vi "Main Output Messages.vi"(8 "error in (no error)":errorcluster, 11 "J1939 Main Configuration":T1={"Parameters"={"J1939 XNET Settings"={"XNET Database"="", "XNET Cluster"="", "CAN Port"="", "Baud rate [Bd]"=0, "Termination"=0, "Incoming Rate"=0, "Outcoming Rate"=1, "Write Decimation"=1}, "Incoming Single Point Configuraiton"={"Incoming Single Point Frame"={"ID"=[], "Conversion"=[], "Channel Array Positions"=[], "Frame Length"=[]}, "Channel Pairs"={"Chan Refs"=[], "Previous Chan Values"=[]}, "Read FIFO"=refnum}, "Outgoing Cyclic Configuraiton"={"Outgoing Cyclic Frame"={"ID"=[], "Conversion"=[], "Channel Array Positions"=[], "Frame Length"=[], "Transmit Propreties"=[]}, "Channel Pairs"={"Block Data Refs"=[], "Previous Chan Values"=[]}, "Write FIFO"=refnum}, "J1939 Monitor Settings"={"J1939 Network Address"=0, "Name"=0}, "Simulated Addresses"=[], "Simulated Addresses LUT"=variant, "Name"=""}, "Name"="", "J1939 Cluster"={"Processed Incoming"=refnum, "Current Device Address"=0, "Processed Outgoing"=refnum, "Process Outgoing"=refnum, "Name"=0}, "References"={"BAM Buffer"=refnum, "CM Buffer"=refnum, "CM Gen"=refnum, "BAM Gen"=refnum, "Address Claims"=refnum, "RQST"=refnum}, "Frame In"="", "Frame Out"="", "Incoming Timeout"=0, "Outgoing Timeout"=0, "Listener ID"=refnum, "Process"=refnum, "Data Ref"=refnum, "Scale Ref"=refnum, "Incoming Direct Access"={"Offset"=0, "Length"=0}, "Outgoing Direct Access"={"Offset"=0, "Length"=0}, "TCP Mngr Ref"=refnum, "Name and Address"="", "Simulated Addresses"=[], "Simulated Addresses LUT"=variant} {"Simulated Addresses"."Simulated Addresses"."J1939 XNET Settings"."Name" format="%.0x"; "Simulated Addresses"."Simulated Addresses"."DM1 Data"."Data Reference" format="%.0x"; "Simulated Addresses"."Simulated Addresses"."DM1 Enable?"."Data Reference" format="%.0x"; "Simulated Addresses"."Simulated Addresses"."DM2 Data"."Data Reference" format="%.0x"; "Simulated Addresses"."Simulated Addresses"."DM2 Enable?"."Data Reference" format="%.0x"; "Parameters"."Simulated Addresses"."Simulated Addresses"."J1939 XNET Settings"."Name" format="%.0x"; "Parameters"."J1939 Monitor Settings"."Name" format="%.0x"; "Parameters"."Outgoing Cyclic Configuraiton"."Channel Pairs"."Block Data Refs"."Data Reference" format="%.0x"; "Parameters"."Outgoing Cyclic Configuraiton"."Outgoing Cyclic Frame"."Transmit Propreties"."Transmit Time" format="%#_p"; "Parameters"."J1939 XNET Settings"."Termination" items=["Off", "On"]; "Parameters"."Incoming Single Point Configuraiton"."Channel Pairs"."Chan Refs" format="%.0x"}) -> (0 "error out":errorcluster)   [LabVIEW 2015, in "J1939 Addon Engine.lvlib"]
uses:
  J1939 Addon Engine.lvlib
  Types/Configuration Cluster.ctl
  <vilib>/NI/NI VeriStand Inline Async API/_VS Inline Async API/Process/Process.lvclass
  Types/Process Parameters.ctl
  Shared/Types/XNET Settings.ctl
  Types/Incoming Single Point Configuration.ctl
  Types/Incoming Single Point Frame Pairs.ctl
  Types/Incoming Single Point Channel Pairs.ctl
  <vilib>/NI Veristand/Custom Device API/Data Reference.ctl
  Types/Outgoing Cyclic Configuration.ctl
  Types/Outgoing Cyclic Frame Pairs.ctl
  Shared/Types/XNET Frame Event Properties.ctl
  Types/Outgoing Cyclic Channel Pairs.ctl
  <vilib>/NI Veristand/Custom Device API/Block Data Reference.ctl
  Shared/Types/Monitor Settings.ctl
  Types/Simulated Settings.ctl
  Shared/Types/Compiled Simulated Settings.ctl
  Types/DTC FIFOs.ctl
  Shared/J1939 Multi Packet Frame/Types/Setup Information Cluster.ctl
  <vilib>/xnet/xnet.llb/XNET Frame CAN.ctl
  <vilib>/xnet/xnet.llb/XNET Frame Type CAN.ctl
  Shared/J1939 Utilities/Types/CAN Outgoing Message Cluster.ctl
  Shared/J1939 Multi Packet Frame/Types/TP List References.ctl
  Shared/J1939 Multi Packet Frame/Types/BAM Buffer Connections List_Ref.ctl
  Shared/J1939 Multi Packet Frame/Types/TP Buffer Connection Cluster.ctl
  Shared/J1939 Multi Packet Frame/Types/Connection Mode Generation Connection Ref.ctl
  Shared/J1939 Multi Packet Frame/Types/Connection Mode Generation Connection Cluster.ctl
  Shared/J1939 Multi Packet Frame/Types/BAM Generation Connections List_Ref.ctl
  Shared/J1939 Multi Packet Frame/Types/BAM Generation Connection Cluster.ctl
  Shared/J1939 Multi Packet Frame/Types/Address Table Reference.ctl
  Shared/J1939 Multi Packet Frame/Types/RQST Lookup Table Reference.ctl
  Types/Data Lookup Table Reference.ctl
  Types/Datatable Lookup DVR.ctl
  Types/Conversion Lookup Table Reference.ctl
  Shared/J1939 Multi Packet Frame/Types/RQST Comm Lookup Table_Ref.ctl
  Shared/STM/Connection Manager/stm_ManagerStateVariables.ctl
  Shared/STM/TCP/stm_TCP Connection Info.ctl
  Shared/STM/_SubVIs/stm_MetaDataElement.ctl
  Shared/STM/Connection Manager/stm_TCPConnectionProperties.ctl
  <vilib>/NI/NI VeriStand Inline Async API/_VS Inline Async API/Process/Process.lvclass/Process.ctl
  <vilib>/NI/NI VeriStand Inline Async API/_VS Inline Async API/Error Handling Process/SubVIs/Error.ConvertArray.vi
  <vilib>/xnet/xnet.llb/XNET Write (Frame CAN).vi
  Shared/J1939 Utilities/J1939 Utilities.lvlib
  <vilib>/NI Veristand/Custom Device API/Custom Device API.lvlib
  Shared/J1939 Addon Shared.lvlib
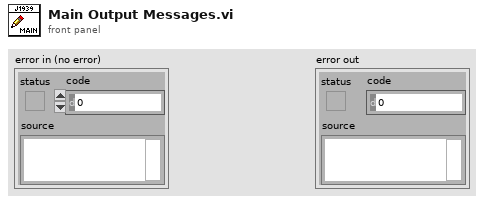
[diagram p1: front panel]
types:
  T1 = typedef "J1939 Addon Engine.lvlib/Configuration Cluster.ctl" = cluster{"Parameters":T2, "Name":string, "J1939 Cluster":T17, "References":T18, "Frame In":refnum<k21>, "Frame Out":refnum<k21>, "Incoming Timeout":u32, "Outgoing Timeout":u32, "Listener ID":refnum<k5>, "Process":refnum<class "Process.lvclass">, "Data Ref":T24, "Scale Ref":T25, "Incoming Direct Access":cluster{"Offset":u32, "Length":u32}, "Outgoing Direct Access":cluster{"Offset":u32, "Length":u32}, "TCP Mngr Ref":T26, "Name and Address":string, "Simulated Addresses":T14[], "Simulated Addresses LUT":variant}
  T2 = typedef "J1939 Addon Engine.lvlib/Process Parameters.ctl" = cluster{"J1939 XNET Settings":T3, "Incoming Single Point Configuraiton":T4, "Outgoing Cyclic Configuraiton":T8, "J1939 Monitor Settings":T13, "Simulated Addresses":T14[], "Simulated Addresses LUT":variant, "Name":string}
  T3 = typedef "J1939 Addon Shared.lvlib/XNET Settings.ctl" = cluster{"XNET Database":refnum<k21>, "XNET Cluster":refnum<k21>, "CAN Port":string, "Baud rate [Bd]":u32, "Termination":u32, "Incoming Rate":u32, "Outcoming Rate":u32, "Write Decimation":u32}
  T4 = typedef "J1939 Addon Engine.lvlib/Incoming Single Point Configuration.ctl" = cluster{"Incoming Single Point Frame":T5, "Channel Pairs":T6, "Read FIFO":refnum<k33>}
  T5 = typedef "J1939 Addon Engine.lvlib/Incoming Single Point Frame Pairs.ctl" = cluster{"ID":u32[], "Conversion":refnum<k21>[], "Channel Array Positions":cluster{"Offset":u32, "Length":u32}[], "Frame Length":u32[]}
  T6 = typedef "J1939 Addon Engine.lvlib/Incoming Single Point Channel Pairs.ctl" = cluster{"Chan Refs":T7[], "Previous Chan Values":dbl[]}
  T7 = typedef "Custom Device API.lvlib/Data Reference.ctl" = i32
  T8 = typedef "J1939 Addon Engine.lvlib/Outgoing Cyclic Configuration.ctl" = cluster{"Outgoing Cyclic Frame":T9, "Channel Pairs":T11, "Write FIFO":refnum<k33>}
  T9 = typedef "J1939 Addon Engine.lvlib/Outgoing Cyclic Frame Pairs.ctl" = cluster{"ID":u32[], "Conversion":refnum<k21>[], "Channel Array Positions":cluster{"Offset":u32, "Length":u32}[], "Frame Length":u32[], "Transmit Propreties":T10[]}
  T10 = typedef "J1939 Addon Shared.lvlib/XNET Frame Event Properties.ctl" = cluster{"Transmit trigger":enum16{"Channel value change"}, "Enable software cyclic trigger":bool, "Transmit Time":dbl}
  T11 = typedef "J1939 Addon Engine.lvlib/Outgoing Cyclic Channel Pairs.ctl" = cluster{"Block Data Refs":T12[], "Previous Chan Values":dbl[]}
  T12 = typedef "Custom Device API.lvlib/Block Data Reference.ctl" = cluster{"Data Reference":T7, "Offset":u64, "Length":u64}
  T13 = typedef "J1939 Addon Shared.lvlib/Monitor Settings.ctl" = cluster{"J1939 Network Address":u8, "Name":u64}
  T14 = typedef "J1939 Addon Engine.lvlib/Simulated Settings.ctl" = cluster{"Simulated Addresses":T15, "FIFOs":T16}
  T15 = typedef "J1939 Addon Shared.lvlib/Compiled Simulated Settings.ctl" = cluster{"J1939 XNET Settings":T13, "DM1 Data":T12[], "DM1 Data":dbl[], "DM1 Enable?":T12[], "DM1 Enable?":dbl[], "DM2 Data":T12[], "DM2 Data":dbl[], "DM2 Enable?":T12[], "DM2 Enable?":dbl[]}
  T16 = typedef "J1939 Addon Engine.lvlib/DTC FIFOs.ctl" = cluster{"DM1 Data":refnum<k33>, "DM1 Enable?":refnum<k33>, "DM2 Data":refnum<k33>, "DM2 Enable?":refnum<k33>, "DM1 Reset?":refnum<k33>, "DM2 Reset?":refnum<k33>}
  T17 = typedef "J1939 Addon Engine.lvlib/Setup Information Cluster.ctl" = cluster{"Processed Incoming":refnum<queue>, "Current Device Address":u8, "Processed Outgoing":refnum<queue>, "Process Outgoing":refnum<queue>, "Name":u64}
  T18 = typedef "J1939 Addon Engine.lvlib/TP List References.ctl" = cluster{"BAM Buffer":T19, "CM Buffer":T19, "CM Gen":T20, "BAM Gen":T21, "Address Claims":T22, "RQST":T23}
  T19 = typedef "J1939 Addon Engine.lvlib/BAM Buffer Connections List_Ref.ctl" = refnum<data-value>
  T20 = typedef "J1939 Addon Engine.lvlib/Connection Mode Generation Connection Ref.ctl" = refnum<data-value>
  T21 = typedef "J1939 Addon Engine.lvlib/BAM Generation Connections List_Ref.ctl" = refnum<data-value>
  T22 = typedef "J1939 Addon Engine.lvlib/Address Table Reference.ctl" = refnum<data-value>
  T23 = typedef "J1939 Addon Engine.lvlib/RQST Lookup Table Reference.ctl" = refnum<data-value>
  T24 = typedef "J1939 Addon Engine.lvlib/Data Lookup Table Reference.ctl" = refnum<data-value>
  T25 = typedef "J1939 Addon Engine.lvlib/Conversion Lookup Table Reference.ctl" = refnum<data-value>
  T26 = typedef "J1939 Addon Engine.lvlib/RQST Comm Lookup Table_Ref.ctl" = refnum<data-value>
  T27 = typedef "J1939 Addon Shared.lvlib/J1939 Utilities.lvlib/CAN Outgoing Message Cluster.ctl" = cluster{"Identifier":u32, "Data":u8[]}
  T28 = typedef "XNET Frame CAN.ctl" = cluster{"timestamp":timestamp, "payload":u8[], "identifier":u32, "type":T29, "extended?":bool, "echo?":bool}
  T29 = typedef "XNET Frame Type CAN.ctl" = u8
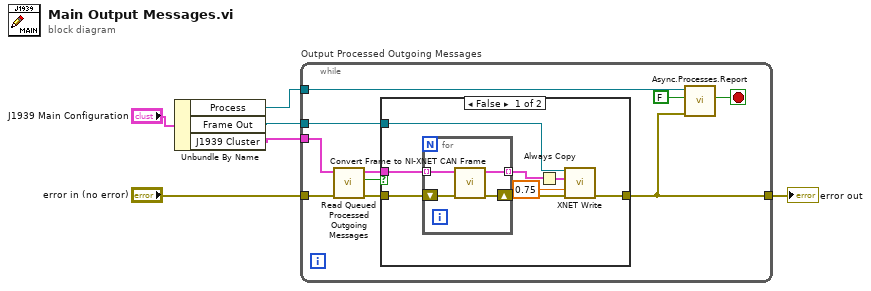
[diagram p0: block diagram]
diagram:
  n1 = Unbundle By Name("J1939 Main Configuration") -> ("Process"=w6:refnum<class "Process.lvclass">, "Frame Out"=w5:refnum<k21>, "J1939 Cluster"=w4:T17)
  n2 = while "Output Processed Outgoing Messages" {
    tunnel: w4 -> [w13]
    tunnel: "error in (no error)" -> [w12]
    tunnel: [w7] -> w1
    tunnel: w5 -> [w9]
    tunnel: w6 -> [w14]
    stop <- w16 stop-if-true
    n3 = call "Read Queued Processed Outgoing Messages.vi"("error in (no error)"=w12, "J1939 Cluster"=w13) -> ("error out"=w11:errorcluster, "timed out?"=w8:bool, "Frames"=w10:T27[])  [unwired: 7 in]
    n4 = case shown="False" w8 {
      tunnel: w11 -> [w24 w29]
      tunnel: w10 -> [w23 _]
      tunnel: w9 -> [w22 _]
      tunnel: [w21 w29] -> w7
      frame False {
        n5 = for {
          tunnel: w23 -> [w26] mode=indexing
          shift-right: [w28] -> w19
          shift-left: w24 -> [w27]
          tunnel: [w25] -> w20 mode=indexing
          n6 = call "Convert Frame to NI-XNET CAN Frame.vi"("error in (no error)"=w27, "Data to Send"=w26) -> ("error out"=w28:errorcluster, "CAN frame"=w25:T28)  [unwired: 8 out]
        }
        n7 = Always Copy(1:w20) -> (0:w17:T28[])
        n8 = call-poly <vilib>:"XNET Write.vi"("session in"=w22, "data"=w17, "timeout (10)"=0.75, "error in (no error)"=w19) -> ("error out"=w21:errorcluster)  [unwired: 11 out]
      }
      frame True {
      }
    }
    n9 = call <vilib>:"Async.Processes.Report.vi"("Error"=w7, "Stop on Error?"=FALSE, "Process in"=w14) -> ("Stop"=w16:bool)  [unwired: 7 in, 1 out]
  }
  "error out" <- w1
